vi "Enqueue Multiple.vi"(0 "State":string[](array[string]), 5 "Data":variant[](array[variant]), 11 "error in (no error)":errorcluster) -> (15 "error out":errorcluster)   [LabVIEW 2014, in "Coding Platform.lvlib"]
uses:
  Coding Platform.lvlib
  Typedefs/Queue Driver Operations.ctl
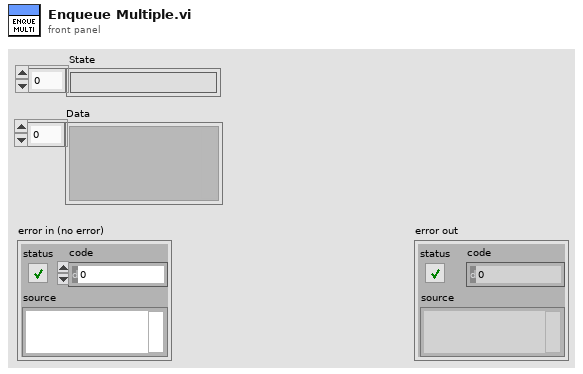
[diagram p1: front panel]
types:
  T1 = typedef "Coding Platform.lvlib/Queue Driver Operations.ctl" = enum16{"Create", "Enqueue", "Dequeue", "Destory"}
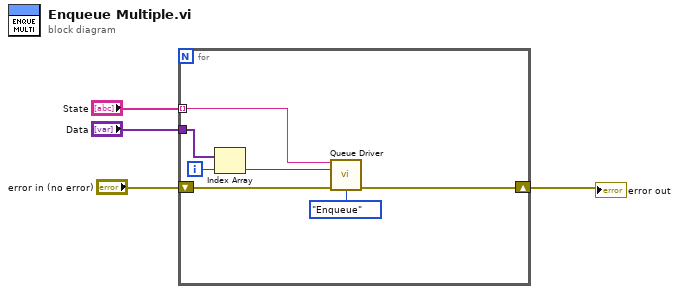
[diagram p0: block diagram]
diagram:
  n1 = for {
    tunnel: "State" -> [w10] mode=indexing
    tunnel: "Data" -> [w7]
    shift-right: [w8] -> w1
    shift-left: "error in (no error)" -> [w9]
    i -> [w5]
    n2 = Index Array(array=w7, index=w5) -> (element=w6:variant)
    n3 = call "Queue Driver.vi"("State"=w10, "Data"=w6, "error in (no error)"=w9, "Operation"=Queue_Driver_Operations."Enqueue") -> ("error out"=w8:errorcluster)  [unwired: 9 in, 2 out]
  }
  "error out" <- w1
